vi "Write Line to Console.vi"(8 "error in (no error)":errorcluster, 10 "Line to Write":string, 11 "Console Ref In":refnum<vi>) -> (0 "error out (no error)":errorcluster, 3 "Console Ref In Out":refnum<vi>)   [LabVIEW 2015]
doc: "Writes a line of text to the string indicator used as a console for target configuration."
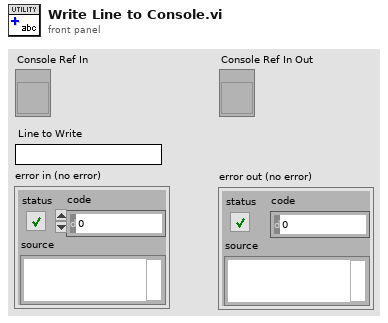
[diagram p1: front panel]
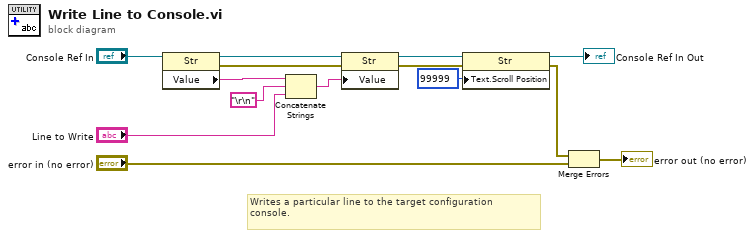
[diagram p0: block diagram]
diagram:
  # "Writes a particular line to the target configuration\nconsole."
  n1 = property class="Str"(reference="Console Ref In") -> (reference out=w10:refnum<vi>, error out=w9:errorcluster, "Value"=w13:string)  [unwired: 1 in]
  n2 = Concatenate Strings(w13, "\r\n", "Line to Write") -> (w8:string)
  n3 = property class="Str"(reference=w10, error in=w9, "Value"=w8) -> (reference out=w5:refnum<vi>, error out=w4:errorcluster)
  n4 = property class="Str"(reference=w5, error in=w4, "Text.Scroll Position"=u32 99999) -> (reference out=→"Console Ref In Out":refnum<vi>, error out=w1:errorcluster)
  n5 = Merge Errors(w1, "error in (no error)") -> (→"error out (no error)":errorcluster)
